vi "encodeObject.vi"(6 "MsgPack Config":T1={"Cluster Conversion"=enum."to array", "Enum Conversion"=enum."to uint", "Use ArrayType"=FALSE}, 8 "error in (no error)":errorcluster, 10 "Variant":variant) -> (0 "error out":errorcluster, 2 "Array":u8[](array[numeric]) format="%.0x")   [LabVIEW 2016, in "MsgPack.lvlib"]
uses:
  MsgPack.lvlib
  SubVis/msgpack_config.ctl
  SubVis/cluster_conversion.ctl
  SubVis/enum_conversion.ctl
  <vilib>/Utility/error.llb/Error Cluster From Error Code.vi
  <vilib>/ErrorRing/Error Ring.xnode
  <vilib>/Utility/Data Type/NI_Data Type.lvlib
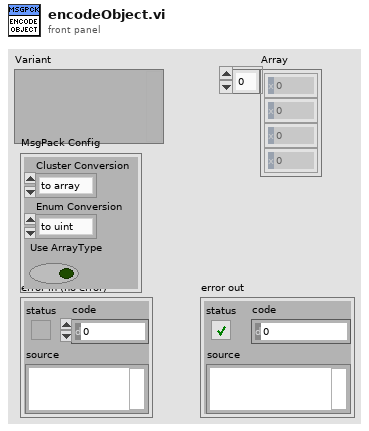
[diagram p1: front panel]
types:
  T1 = typedef "MsgPack.lvlib/msgpack_config.ctl" = cluster{"Cluster Conversion":T2, "Enum Conversion":T3, "Use ArrayType":bool}
  T2 = typedef "MsgPack.lvlib/cluster_conversion.ctl" = enum16{"to map", "to array"}
  T3 = typedef "MsgPack.lvlib/enum_conversion.ctl" = enum16{"to uint", "to string"}
  T4 = typedef "NI_Data Type.lvlib/Data Type.ctl" = enum8{"Invalid Type", "Void", "I8", "I16", "I32", "I64", "U8", "U16", "U32", "U64", "Single Float", "Double Float", "Extended Float", "Single Complex", "Double Complex", "Extended Complex", "Enum U8", "Enum U16", "Enum U32", "Enum U64", "Single Float With Unit", "Double Float With Unit", "Extended Float With Unit", "Single Complex with Unit", "Double Complex with Unit", "Extended Complex with Unit", "Boolean", "String", "Path", "Picture", "Tag", "Array", "Cluster", "Variant", "LV Variant", "Waveform", "Timestamp", "Digital Waveform", "Digital Data", "ExpressData", "Refnum", "External Data", "VI", "Poly VI", "LabVIEW Class Instance", "Fixed Point"}
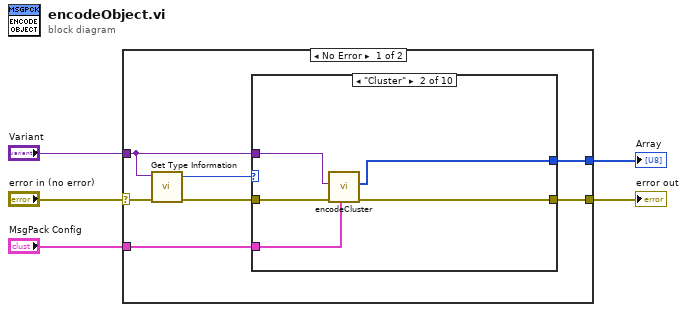
[diagram p0: block diagram]
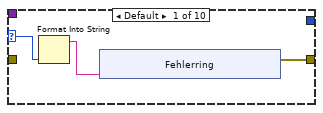
[diagram p2: hidden frame]
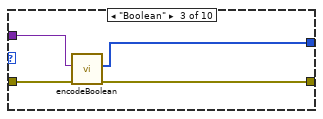
[diagram p3: hidden frame]
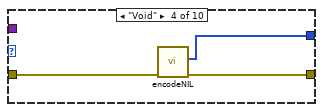
[diagram p4: hidden frame]
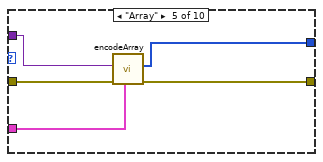
[diagram p5: hidden frame]
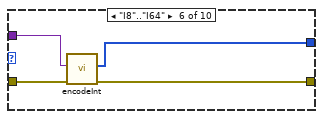
[diagram p6: hidden frame]
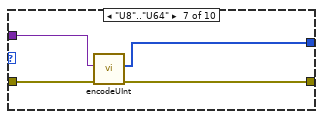
[diagram p7: hidden frame]
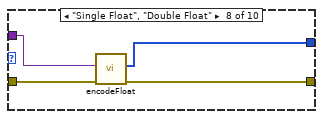
[diagram p8: hidden frame]
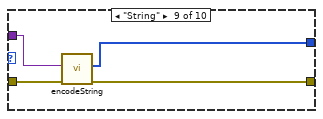
[diagram p9: hidden frame]
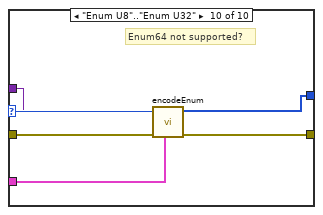
[diagram p10: hidden frame]
diagram:
  n1 = case shown="No Error" "error in (no error)" {
    selector: "error in (no error)" -> [w8 w62]
    tunnel: "Variant" -> [w11 _]
    tunnel: [w10 w62] -> w4
    tunnel: [w9 _] -> w3
    tunnel: "MsgPack Config" -> [w6 _]
    frame No Error {
      n2 = call <vilib>:"Get Type Information.vi"("error in (no error)"=w8, "Variant"=w11) -> ("error out"=w12:errorcluster, "Type"=w7:T4)  [unwired: 5 in, 3 out]
      n3 = case shown="\"Cluster\"" w7 {
        selector: w7 -> [w14 _ _ _ _ _ _ _ _ w58]
        tunnel: w12 -> [_ w27 w31 w34 w39 w43 w47 w51 w55 w59]
        tunnel: w11 -> [_ w26 w28 _ w38 w42 w46 w50 w54 w57]
        tunnel: [w15 w25 w30 w33 w36 w40 w45 w48 w52 w61] -> w10
        tunnel: [_ w24 w29 w32 w37 w41 w44 w49 w53 w60] -> w9
        tunnel: w6 -> [_ w23 _ _ w35 _ _ _ _ w56]
        frame Default {
          n4 = Format Into String(w14) -> (resulting string=w13:string)  [unwired: 3 in, 1 out]
          n5 = xnode "Fehlerring"("parameter 0"=w13) -> ("error out"=w15:errorcluster)
        }
        frame "Cluster" {
          n6 = call "encodeCluster.vi"("MsgPack Config"=w23, "error in (no error)"=w27, "Variant"=w26) -> ("error out"=w25:errorcluster, "Array"=w24:u8[])  [unwired: 7 in]
        }
        frame "Boolean" {
          n7 = call "encodeBoolean.vi"("error in (no error)"=w31, "Variant"=w28) -> ("error out"=w30:errorcluster, "Array"=w29:u8[])  [unwired: 8 in]
        }
        frame "Void" {
          n8 = call "encodeNIL.vi"("error in (no error)"=w34) -> ("error out"=w33:errorcluster, "Array"=w32:u8[])  [unwired: 9 in]
        }
        frame "Array" {
          n9 = call "encodeArray.vi"("MsgPack Config"=w35, "error in (no error)"=w39, "Variant"=w38) -> ("error out"=w36:errorcluster, "Array"=w37:u8[])  [unwired: 7 in]
        }
        frame "I8".."I64" {
          n10 = call "encodeInt.vi"("error in (no error)"=w43, "Variant"=w42) -> ("error out"=w40:errorcluster, "Array"=w41:u8[])  [unwired: 8 in]
        }
        frame "U8".."U64" {
          n11 = call "encodeUInt.vi"("error in (no error)"=w47, "Variant"=w46) -> ("error out"=w45:errorcluster, "Array"=w44:u8[])  [unwired: 8 in]
        }
        frame "Single Float", "Double Float" {
          n12 = call "encodeFloat.vi"("error in (no error)"=w51, "Variant"=w50) -> ("error out"=w48:errorcluster, "Array"=w49:u8[])  [unwired: 8 in]
        }
        frame "String" {
          n13 = call "encodeString.vi"("error in (no error)"=w55, "Variant"=w54) -> ("error out"=w52:errorcluster, "Array"=w53:u8[])  [unwired: 8 in]
        }
        frame "Enum U8".."Enum U32" {
          # "Enum64 not supported?"
          n14 = call "encodeEnum.vi"("MsgPack Config"=w56, "error in (no error)"=w59, "Type"=w58, "Variant"=w57) -> ("error out"=w61:errorcluster, "Array"=w60:u8[])  [unwired: 6 in]
        }
      }
    }
    frame Error {
    }
  }
  "Array" <- w3
  "error out" <- w4
